vi "Set Powerline Frequency Parameter.vi"(8 "error in (no error)":errorcluster, 10 "Value":i32, 11 "Stream in":refnum<class "Stream.lvclass">) -> (0 "error out":errorcluster, 1 "Set Value":i32, 3 "Stream":refnum<class "Stream.lvclass">)   [LabVIEW 2020, in "capture.lvlib" / "Stream.lvclass"]
doc: "Set Powerline Frequency Parameter."
uses:
  Stream.lvclass
  Camera Parameters.ctl
  Stream.lvclass/Stream.ctl
  <vilib>/Utility/error.llb/Error Cluster From Error Code.vi
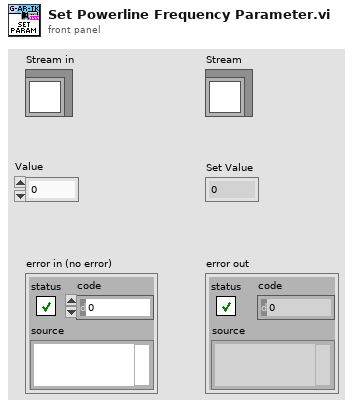
[diagram p1: front panel]
types:
  T1 = typedef "capture.lvlib/Stream.lvclass/Camera Parameters.ctl" = enum8{"EXPOSURE", "FOCUS", "ZOOM", "GAIN", "WHITE_BALANCE_TEMPERATURE", "BRIGHTNESS", "CONTRAST", "SATURATION", "GAMMA", "HUE", "SHARPNESS", "BACKLIGHT_COMPENSATION", "POWER_LINE_FREQUENCY"}
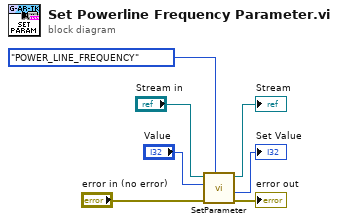
[diagram p0: block diagram]
diagram:
  n1 = call "SetParameter.vi"("Camera Parameter"=Camera_Parameters."POWER_LINE_FREQUENCY", "error in (no error)"="error in (no error)", "Value"="Value", "Stream in"="Stream in") -> ("error out"=→"error out":errorcluster, "Set Value"=→"Set Value":i32, "Stream"=→"Stream":refnum<class "Stream.lvclass">)  [unwired: 5 in]
